vi "test_LogFile Exists on Target.vi"(8 "error in (no error)":errorcluster, 11 "TestCase in":refnum<class "Telemetry System Tests.lvclass">) -> (0 "error out":errorcluster, 3 "TestCase out":refnum<class "Telemetry System Tests.lvclass">)   [LabVIEW 2019, in "Telemetry System Tests.lvclass"]
uses:
  Telemetry System Tests.lvclass
  4c642fb7-04a0-4729-a002-4e235dd1b0d8.vi
  <vilib>/addons/_JKI Toolkits/VI Tester/TestCase.llb/TestCase.lvclass
  TLCD Test/TLCD Test.lvclass
  C:/Program Files (x86)/National Instruments/LabVIEW 2019/vi.lib/addons/_JKI Toolkits/VI Tester/TestCase.llb/TestCase.lvclass
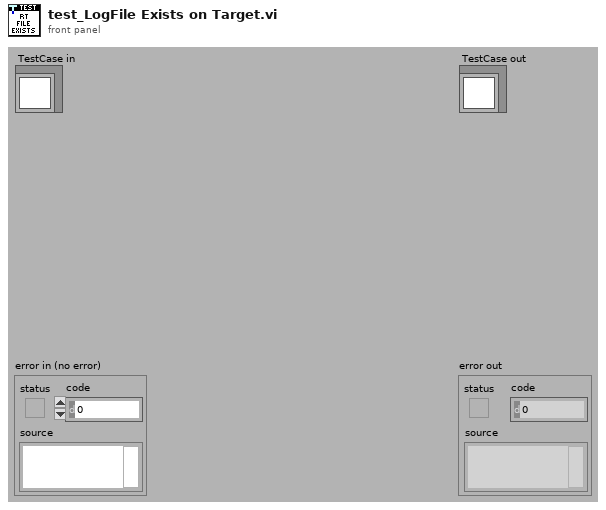
[diagram p1: front panel]
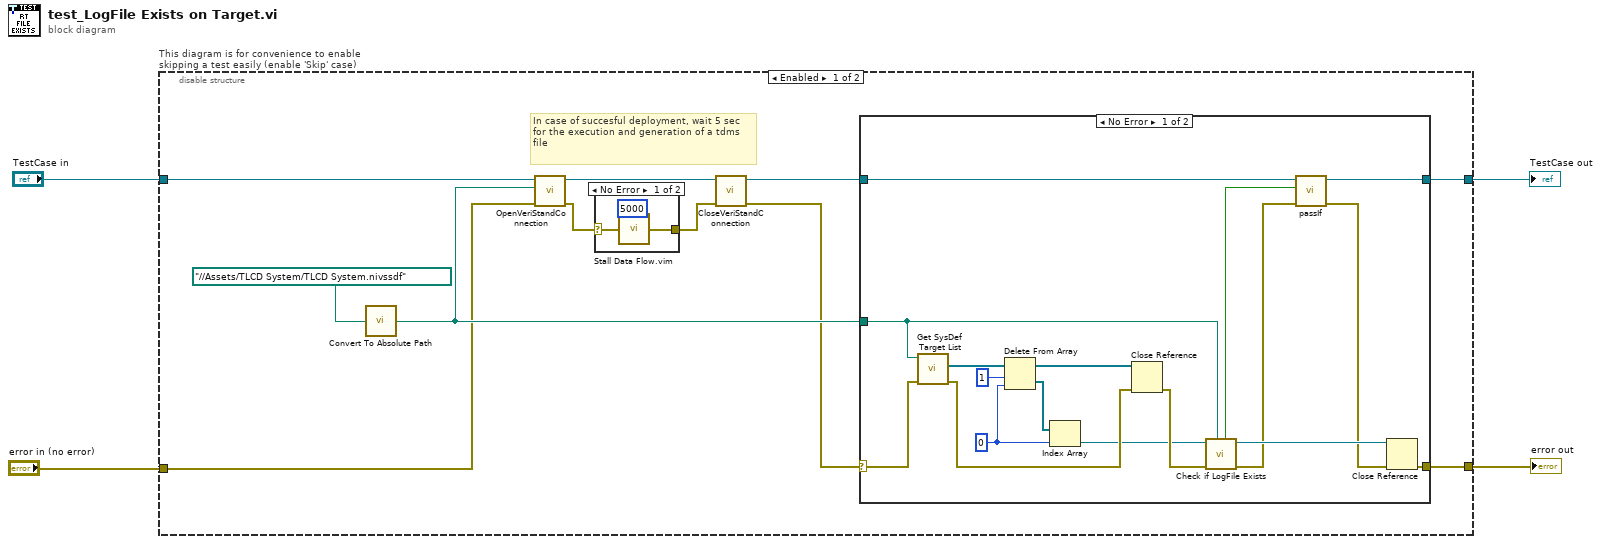
[diagram p0: block diagram]
diagram:
  n1 = disable-structure "This diagram is for convenience to enable skipping a test easily (enable 'Skip' case)" shown="Enabled" {
    disable-tunnel: "TestCase in" -> [w12 w42]
    disable-tunnel: [w13 w40] -> w1
    disable-tunnel: [w14 w41] -> w3
    disable-tunnel: "error in (no error)" -> [w9 w39]
    frame Enabled {
      # "In case of succesful deployment, wait 5 sec for the execution and generation of a tdms file"
      n2 = call "Convert To Absolute Path.vi"("System Definition File Path"=path "../../Assets/TLCD System/TLCD System.nivssdf" ("relative base path")) -> ("Absolute path"=w10:path)
      n3 = call-dynamic "OpenVeriStandConnection.vi"("error in (no error)"=w9, "System Definition File"=w10, "VeriStand Test Case in"=w12) -> ("error out"=w6:errorcluster, "VeriStand Test Case out"=w7:refnum<class "Telemetry System Tests.lvclass">)  [unwired: 6 in, 1 out]
      n4 = case shown="No Error" w6 {
        selector: w6 -> [w18 w19]
        tunnel: [w16 w19] -> w5
        frame No Error {
          n5 = call "Stall Data Flow.vim"("value in"=w18, "milliseconds to wait"=u32 5000) -> ("value out"=w16:errorcluster)  [unwired: 1 out]
        }
        frame Error {
        }
      }
      n6 = call-dynamic "CloseVeriStandConnection.vi"("error in (no error)"=w5, "VeriStand Test Case in"=w7) -> ("error out"=w8:errorcluster, "VeriStand Test Case out"=w11:refnum<class "Telemetry System Tests.lvclass">)  [unwired: 8 in]
      n7 = case shown="No Error" w8 {
        selector: w8 -> [w20 w38]
        tunnel: [w36 w38] -> w14
        tunnel: [w26 w37] -> w13
        tunnel: w11 -> [w22 w37]
        tunnel: w10 -> [w21 _]
        frame No Error {
          w32 = 0 ("index")
          n8 = call "Get SysDef Target List.vi"("error in (no error)"=w20, "System Definition Path"=w21) -> ("error out"=w30:errorcluster, "Target List"=w35:refnum<k24>[])  [unwired: 8 in]
          n9 = Delete From Array(array=w35, length=1, index=w32) -> (deleted portion=w33:refnum<k24>[], array with subset deleted=w31:refnum<k24>[])
          n10 = Index Array(array=w33, index=w32) -> (element=w27:refnum<k24>)
          n11 = Close Reference(reference=w31, error in (no error)=w30) -> (error out=w28:errorcluster)
          n12 = call "Check if LogFile Exists.vi"("System Definition Path"=w21, "error in (no error)"=w28, "Target Refnum in"=w27) -> ("error out"=w25:errorcluster, "Target Refnum out"=w29:refnum<k24>, "LogFile Exists?"=w23:bool)  [unwired: 6 in]
          n13 = call-dynamic "passIf.vi"("error in (no error)"=w25, "pass"=w23, "TestCase in"=w22) -> ("error out"=w24:errorcluster, "TestCase out"=w26:refnum<class "Telemetry System Tests.lvclass">)  [unwired: 7 in]
          n14 = Close Reference(reference=w29, error in (no error)=w24) -> (error out=w36:errorcluster)
        }
        frame Error {
        }
      }
    }
    frame Disabled {
      # "skip test result while test is under development"
      n15 = call <vilib>:"skip.vi"("error in (no error)"=w39, "TestCase in"=w42) -> ("error out"=w41:errorcluster, "TestCase out"=w40:refnum<class "Telemetry System Tests.lvclass">)  [unwired: 8 in]
    }
  }
  "error out" <- w3
  "TestCase out" <- w1
